vi "Set PublicEvents.vi"(8 "error in (no error)":errorcluster, 10 "Public Events":T1, 11 "Log_Engine in":refnum<class "Log_Engine.lvclass">) -> (0 "error out":errorcluster, 3 "Log_Engine out":refnum<class "Log_Engine.lvclass">)   [LabVIEW 2019, in "Log_Engine.lvclass"]
doc: "Developed by Kevin Thompson\nkevin@thompsonengineering.net\n\nCopyright 2018\nThompson Engineering, LLC"
uses:
  Log_Engine.lvclass
  DataTypes/Public Events--cluster.ctl
  Common/DataTypes/TD Async CmdMsg EventData--cluster.ctl
  DataTypes/LogStateChg EvData--cluster.ctl
  DataTypes/LogStateEvData--cluster.ctl
  Common/DataTypes/LogState--enum.ctl
  DataTypes/TDMSStateChg EvData--cluster.ctl
  DataTypes/TDMSStateEvData--cluster.ctl
  Common/DataTypes/TDMSState--enum.ctl
  Log_Engine.lvclass/Log_Engine.ctl
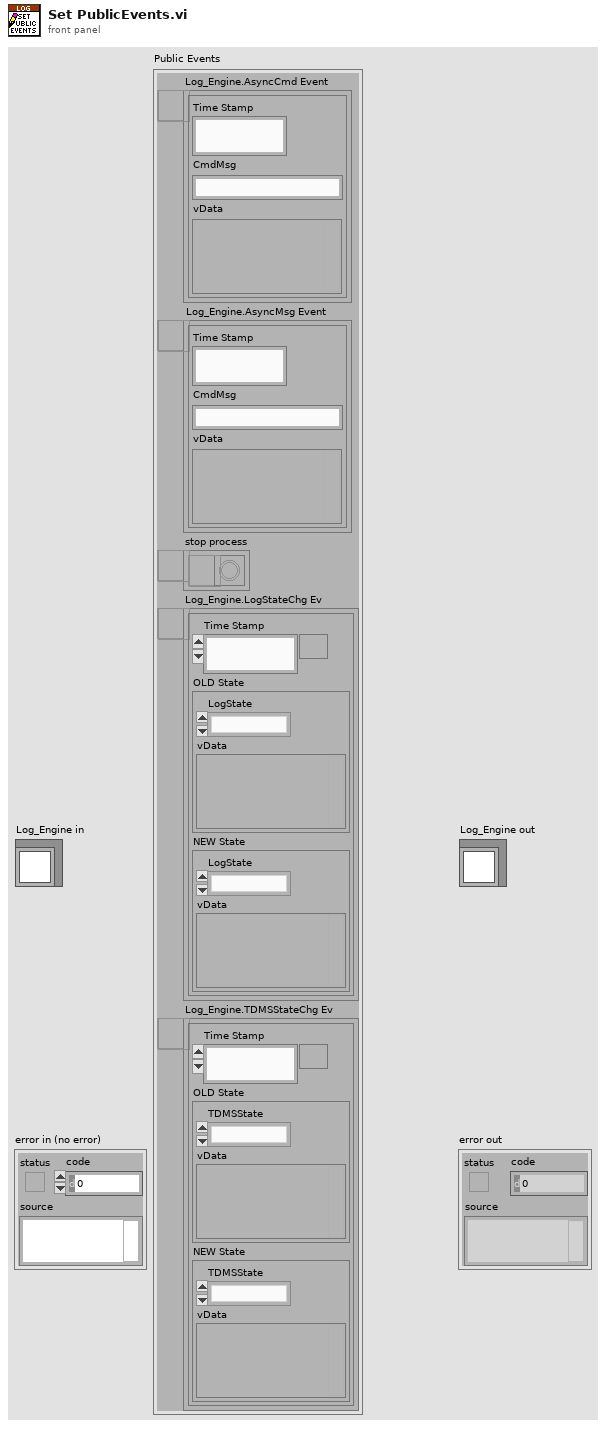
[diagram p1: front panel]
types:
  T1 = typedef "Log_Engine.lvclass/Public Events--cluster.ctl" = cluster{"Log_Engine.AsyncCmd Event":refnum<user-event>, "Log_Engine.AsyncMsg Event":refnum<user-event>, "stop process":refnum<user-event>, "Log_Engine.LogStateChg Ev":refnum<user-event>, "Log_Engine.TDMSStateChg Ev":refnum<user-event>}
  T2 = typedef "Log_Engine.lvclass/ObjData--cluster.ctl" = cluster{"Settings":T3, "Public Events":T1, "Dependency":T4, "ReadData-placeholder":T5, "VISA-placeholder":refnum<visa-resource-name>, "InverterWaveformsQ":T6, "LogState":T7, "TDMSState":T8}
  T3 = typedef "Log_Engine.lvclass/Settings--cluster.ctl" = cluster{"Simulation":bool, "TDMS_FolderPath":string, "CSV_FolderPath":string, "TDMS_FileName_Prefix":string, "CSV_FileName_Prefix":string, "TDMS_LogDuration(s)":dbl, "CSV_LogDuration(s)":dbl}
  T4 = typedef "Log_Engine.lvclass/Dependency--cluster.ctl" = cluster{"Config":refnum<class "Config.lvclass">, "DAQ_Engine":refnum<class "DAQ_Engine.lvclass">}
  T5 = typedef "Log_Engine.lvclass/Read Data--cluster.ctl" = cluster{"Data":dbl}
  T6 = typedef "InverterWaveforms--QRef.ctl" = refnum<queue>
  T7 = typedef "LogState--enum.ctl" = enum16{"Unknown", "Stopped", "Running", "Error"}
  T8 = typedef "TDMSState--enum.ctl" = enum16{"Unknown", "Stopped", "Running", "Error"}
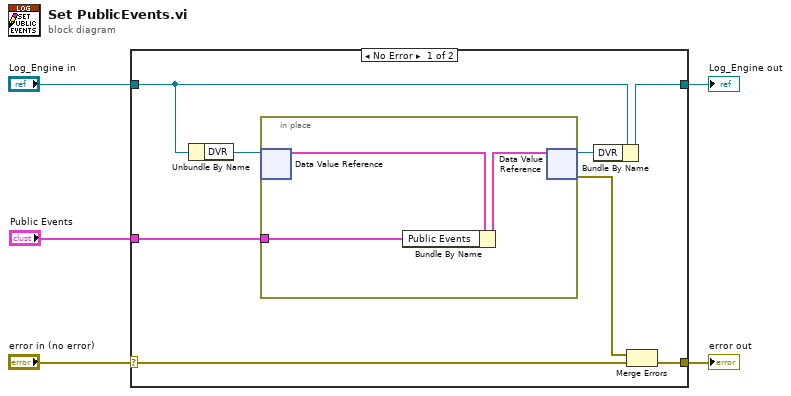
[diagram p0: block diagram]
diagram:
  n1 = case shown="No Error" "error in (no error)" {
    selector: "error in (no error)" -> [w8 w17]
    tunnel: [w6 w17] -> w4
    tunnel: [w7 w18] -> w2
    tunnel: "Log_Engine in" -> [w10 w18]
    tunnel: "Public Events" -> [w9 _]
    frame No Error {
      n2 = Unbundle By Name(w10) -> ("DVR"=w13:refnum<data-value>)
      n3 = in-place {
        in-place-border: w9 -> [w14]
        n4 = in-place-dvr #1(w13) -> (w16:T2)  [unwired: 1 out]
        n5 = Bundle By Name(cluster=w16, "Public Events"=w14) -> (w15:T2)
        n6 = in-place-dvr #1(w15) -> (w12:refnum<data-value>, w11:errorcluster)
      }
      n7 = Bundle By Name(cluster=w10, "DVR"=w12) -> (w7:refnum<class "Log_Engine.lvclass">)
      n8 = Merge Errors(w11, w8) -> (w6:errorcluster)
    }
    frame Error {
    }
  }
  "error out" <- w4
  "Log_Engine out" <- w2
